vi "WPI_DashboardCreate AVI.vi"(8 "Display Name":string, 9 "Recording":u16(ring) items=["O", "*", "Open Playback Panel"], 10 "frames per seconds":u32=30, 11 "Image":T1) -> ()   [LabVIEW 2017]
doc: "Depending on Recording Mode, create or add to an AVI file using the Camera IP as part of the name to distinguish different cameras."
uses:
  <vilib>/vision/Image Controls.llb/IMAQ Image.ctl
  <vilib>/vision/Avi.llb/IMAQ AVI2 Refnum.ctl
  <vilib>/Rock Robotics/WPI/Dashboard/WPI_DashboardLogging Global.vi
panel:
  in  "Rec Mode":u16(ring)
  out "Codec Names":string[](array[string])
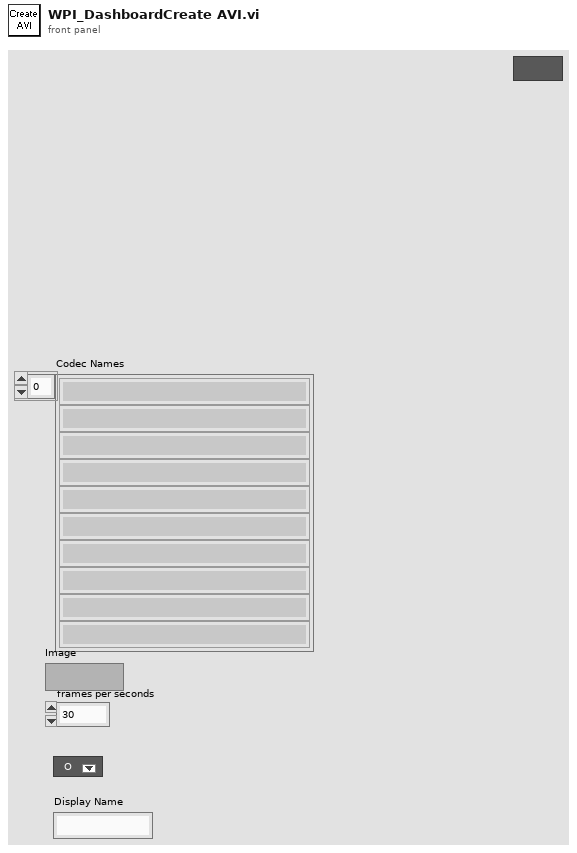
[diagram p1: front panel]
types:
  T1 = typedef "IMAQ Image.ctl" = refnum<image>
  T2 = typedef "IMAQ AVI2 Refnum.ctl" = refnum<k20>
  T3 = cluster{i32, "millisecond timer value":u32, "AVI Refnum (duplicate)":T2, "Display Index":u32}
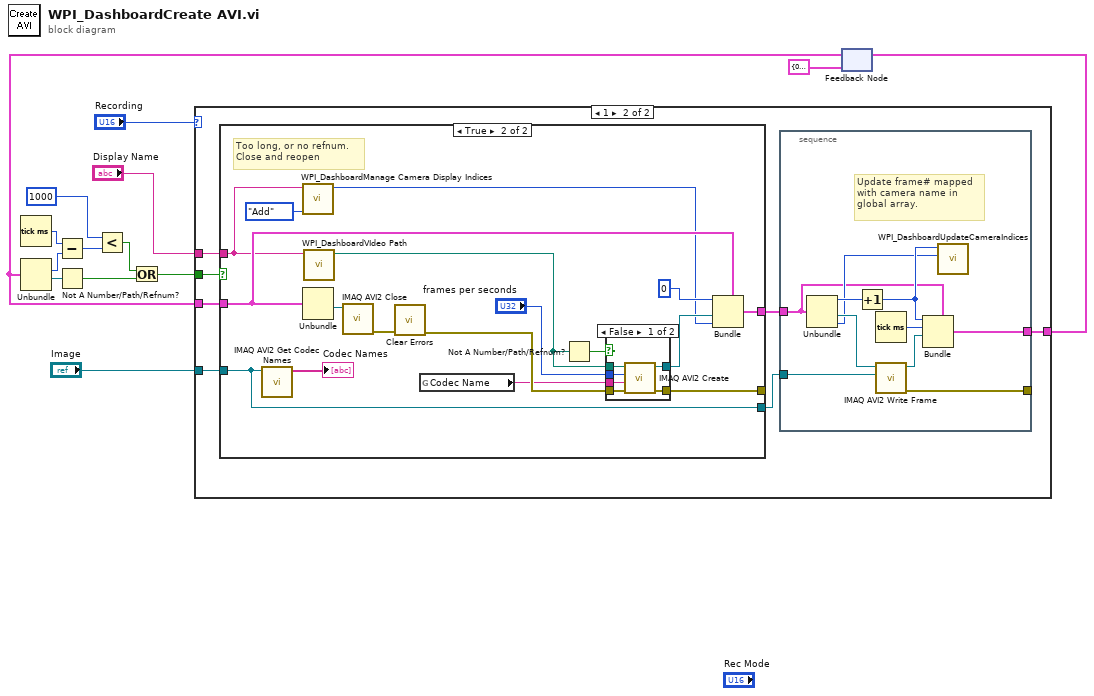
[diagram p0: block diagram]
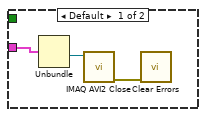
[diagram p2: hidden frame]
diagram:
  n1 = Tick Count (ms)() -> (millisecond timer value=w12:u32)
  n2 = feedback #1(T3 {0, "millisecond timer value"=0, "AVI Refnum (duplicate)"=refnum, "Display Index"=0}) -> (w6:T3)
  n3 = Unbundle(w6) -> ("millisecond timer value"=w2:u32, "AVI Refnum (duplicate)"=w3:T2)  [unwired: 2 out]
  n4 = Subtract(x=w12, y=w2) -> (x-y=w10:u32)
  n5 = Not A Number/Path/Refnum?(number/path/refnum=w3) -> (NaN/Path/Refnum?=w11:bool)
  n6 = Less?(x=1000, y=w10) -> (x < y?=w8:bool)
  n7 = Or(x=w8, y=w11) -> (x .or. y?=w7:bool)
  n8 = case shown="1" "Recording" {
    tunnel: "Image" -> [_ w24]
    tunnel: [_ w22] -> w13
    tunnel: w7 -> [_ w21]
    tunnel: w6 -> [w17 w20]
    tunnel: "Display Name" -> [_ w18]
    frame Default {
      n9 = Unbundle(w17) -> ("AVI Refnum (duplicate)"=w15:T2)  [unwired: 3 out]
      n10 = call "IMAQ AVI2 Close"("AVI Refnum"=w15) -> ("error out"=w16:errorcluster)  [unwired: 10 in]
      n11 = call <vilib>:"Clear Errors.vi"("error in (no error)"=w16) -> ()  [unwired: 5 in, 2 out]
    }
    frame 1 {
      n12 = case shown="True" w21 {
        tunnel: w24 -> [w36 w51]
        tunnel: [w36 w51] -> w23
        tunnel: w20 -> [w35 w48]
        tunnel: [w35 w47] -> w19
        tunnel: w18 -> [_ w39]
        tunnel: [_ w46] -> _
        frame False {
        }
        frame True {
          # "Too long, or no refnum.\nClose and reopen"
          n13 = call "IMAQ AVI2 Get Codec Names"("Image"=w51) -> ("Codec Names"=→"Codec Names":string[])  [unwired: 9 in, 1 out]
          n14 = call <vilib>:"WPI_DashboardManage Camera Display Indices.vi"("Operation"=enum16{"Add", "Retrieve"}."Add", "Display Name"=w39) -> ("index of element"=w38:i32)  [unwired: 9 in]
          n15 = Unbundle(w48) -> ("AVI Refnum (duplicate)"=w43:T2)  [unwired: 3 out]
          n16 = call <vilib>:"WPI_DashboardVIdeo Path.vi"("Camera IP"=w39) -> ("Video Path"=w44:path)  [unwired: 10 in]
          n17 = call "IMAQ AVI2 Close"("AVI Refnum"=w43) -> ("error out"=w50:errorcluster)  [unwired: 10 in]
          n18 = call <vilib>:"Clear Errors.vi"("error in (no error)"=w50) -> ("error out"=w49:errorcluster)  [unwired: 5 in, 1 out]
          n19 = global read "WPI_DashboardLogging Global.vi" "Codec Name"() -> (w40:string)
          n20 = Not A Number/Path/Refnum?(number/path/refnum=w44) -> (NaN/Path/Refnum?=w45:bool)
          n21 = case shown="False" w45 {
            tunnel: w40 -> [w59 _]
            tunnel: "frames per seconds" -> [w58 _]
            tunnel: w49 -> [w57 w60]
            tunnel: [w56 _] -> w42
            tunnel: [w55 w60] -> w46
            tunnel: w44 -> [w54 _]
            frame False {
              n22 = call "IMAQ AVI2 Create"("error in (no error)"=w57, "Codec"=w59, "Frames Per Second"=w58, "AVI Path"=w54) -> ("error out"=w55:errorcluster, "AVI Refnum"=w56:T2)  [unwired: 6 in]
            }
            frame True {
            }
          }
          n23 = Bundle(cluster=w48, 0, "AVI Refnum (duplicate)"=w42, "Display Index"=w38) -> (w47:T3)  [unwired: 1 in]
        }
      }
      n24 = stacked-sequence {
        tunnel: w23 -> [w34]
        tunnel: [w31] -> w22
        tunnel: w19 -> [w25]
        tunnel: [w28] -> _
        frame #0 {
          # "Update frame# mapped\nwith camera name in\nglobal array."
          n25 = Unbundle(w25) -> (w27:i32, "AVI Refnum (duplicate)"=w30:T2, "Display Index"=w26:u32)  [unwired: 1 out]
          n26 = Increment(x=w27) -> (x+1=w29:i32)
          n27 = Tick Count (ms)() -> (millisecond timer value=w33:u32)
          n28 = call "IMAQ AVI2 Write Frame"("Image"=w34, "AVI Refnum"=w30) -> ("error out"=w28:errorcluster, "AVI Refnum (duplicate)"=w32:T2)  [unwired: 7 in, 1 out]
          n29 = Bundle(cluster=w25, w29, "millisecond timer value"=w33, "AVI Refnum (duplicate)"=w32) -> (w31:T3)  [unwired: 1 in]
          n30 = call <vilib>:"WPI_DashboardUpdateCameraIndices.vi"("Display Index"=w26, "Numeric"=w29) -> ()  [unwired: 10 in]
        }
      }
    }
  }
  n31 = feedback-in #1(w13) -> ()
